vi "Actor Core.vi"(8 "error in":errorcluster, 11 "UI Controller in":refnum<class "UI Controller.lvclass">) -> (0 "error out":errorcluster, 3 "Actor out":refnum<class "Actor.lvclass">)   [LabVIEW 2019, in "UI Controller.lvlib" / "UI Controller.lvclass"]
doc: "(<B>Filename</B>: Actor Framework.lvlib:Actor.lvclass:Actor Core.vi)\n\nReceives messages to the actor, reacts to them, and initiates any error handling that may shut the actor down.\n\nDescendant classes may override this VI to append parallel tasks for the actor to complete while it handles messages. Overrides use the Call Parent Method node."
uses:
  UI Controller.lvclass
  C:/Program Files (x86)/National Instruments/LabVIEW 2019/vi.lib/ActorFramework/Actor/Actor.lvclass
  <vilib>/ActorFramework/Actor/Actor.lvclass
  <vilib>/ActorFramework/Actor/Actor.lvclass/Actor.ctl
  <vilib>/ActorFramework/Message Enqueuer/Message Enqueuer.lvclass/Message Enqueuer.ctl
  UI Controller.lvclass/UI Controller.ctl
  <vilib>/ActorFramework/Message Enqueuer/Init from Existing Queue.vi
  <vilib>/ActorFramework/Message Enqueuer/Enqueue.vi
  <vilib>/ActorFramework/Stop Msg/Stop Msg.lvclass
  C:/Program Files (x86)/National Instruments/LabVIEW 2019/vi.lib/ActorFramework/Message/Message.lvclass
  <vilib>/ActorFramework/Message Priority Queue/Priority Enqueue.vi
  <vilib>/ActorFramework/Message Enqueuer/Message Enqueuer.lvclass
  New Event UI/New Event UI/New Event UI.lvclass
  C:/GIT/Event-Diplom/Source/Event Diplom NI-AF/UI Controller/UI Controller/UI Controller.lvclass
panel:
  in  "New Event":bool
  in  "Events":i32(listbox)
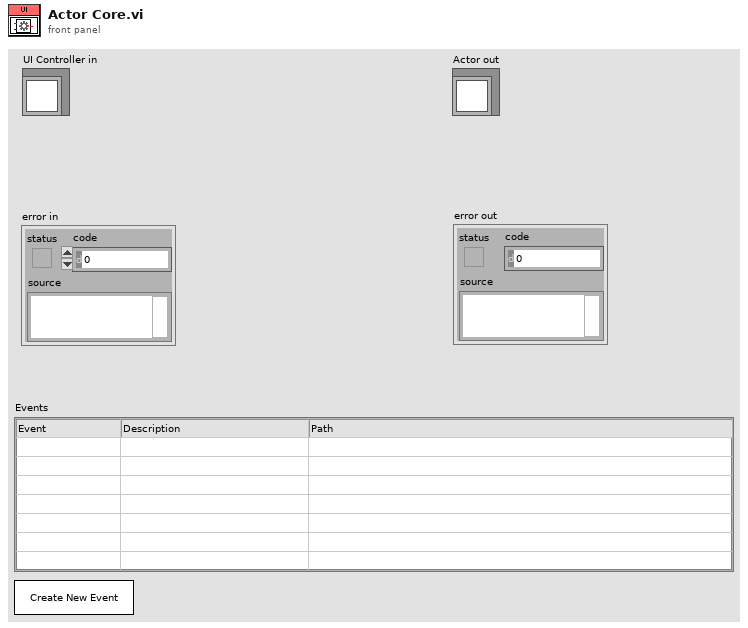
[diagram p1: front panel]
types:
  T1 = enum32{"Invalid", "Standard", "Closed", "Hidden", "Minimized", "Maximized"}
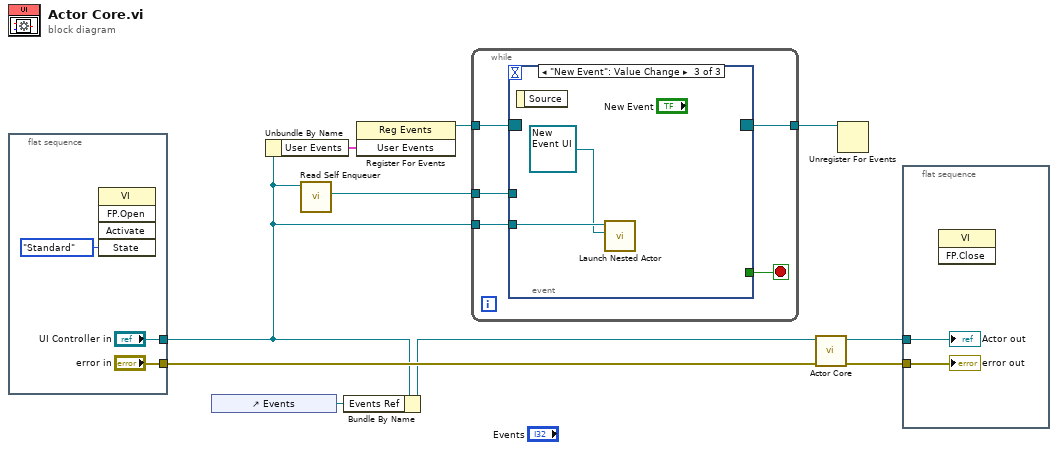
[diagram p0: block diagram]
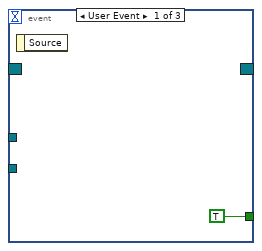
[diagram p2: hidden frame]
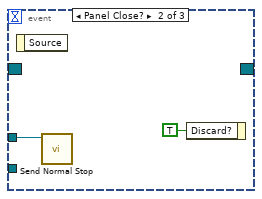
[diagram p3: hidden frame]
diagram:
  n1 = flat-sequence {
    tunnel: ["error in"] -> w8
    tunnel: ["UI Controller in"] -> w1
    frame #0 {
      n2 = invoke class="VI" method="FP.Open"("State"=T1."Standard") -> ()  [unwired: 4 in, 5 out]
    }
  }
  n3 = control-ref of="Events"() -> (w2:refnum<vi>)
  n4 = Unbundle By Name(w1) -> ("User Events"=w7:cluster{"Stop":refnum<user-event>})
  n5 = call <vilib>:"Read Self Enqueuer.vi"("Actor"=w1) -> ("Self Enqueuer"=w4:refnum<class "Message Enqueuer.lvclass">)  [unwired: 10 in]
  n6 = Bundle By Name(cluster=w1, "Events Ref"=w2) -> (w3:refnum<class "UI Controller.lvclass">)
  n7 = register-events(w7) -> (reference out=w6:refnum<event-registration>)  [unwired: 2 in, 1 out]
  n8 = while {
    tunnel: w6 -> [w18]
    tunnel: [w17] -> w5
    tunnel: w4 -> [w15]
    tunnel: w1 -> [w14]
    stop <- w16 stop-if-true
    n9 = event shown="[2] \"New Event\": Value Change" {
      selector: w18 -> [_ _ _]
      dyn-events: [_ _ _] -> w17
      timeout: _ -> [_ _ _]
      tunnel: [TRUE _ _] -> w16
      tunnel: w15 -> [_ w20 _]
      tunnel: w14 -> [_ _ w23]
      event User Event {
        n10 = event-data() -> ()  [unwired: 1 in, 1 out]
      }
      event Panel Close? {
        n11 = event-data() -> ()  [unwired: 1 in, 1 out]
        n12 = call <vilib>:"Send Normal Stop.vi"("Message Enqueuer"=w20) -> ()  [unwired: 10 in, 1 out]
        n13 = event-data("Discard?"=TRUE) -> ()  [unwired: 1 in, 1 out]
      }
      event "New Event": Value Change {
        n14 = event-data() -> ()  [unwired: 1 in, 1 out]
        n15 = call <vilib>:"Launch Nested Actor.vi"("Nested Actor"=refnum<class "New Event UI.lvclass"> refnum ("New Event UI.lvlib:New Event UI.lvclass"), "Caller Actor in"=w23) -> ()  [unwired: 7 in, 3 out]
      }
    }
  }
  n16 = call-parent "Actor Core.vi"("error in"=w8, "Actor in"=w3) -> ("error out"=w10:errorcluster, "Actor out"=w9:refnum<class "Actor.lvclass">)  [unwired: 8 in]
  n17 = Unregister For Events(event registration refnum=w5) -> ()  [unwired: 1 in, 1 out]
  n18 = flat-sequence {
    tunnel: w10 -> [w25]
    tunnel: w9 -> [w24]
    frame #0 {
      n19 = invoke class="VI" method="FP.Close"() -> ()  [unwired: 3 in, 3 out]
      "error out" <- w25
      "Actor out" <- w24
    }
  }
